vi "UpdateLimsTestStepAutomation.vi"(7 "step_id":u32, 8 "error in (no error)":errorcluster, 9 "instruction_automation":string, 10 "link_automation":string, 11 "ByteGSAPIBase in":refnum<class "ByteGSAPIBase.lvclass">) -> (0 "error out":errorcluster, 2 "Result Step":T1, 3 "ByteGSAPIBase out":refnum<class "ByteGSAPIBase.lvclass">)   [LabVIEW 2019, in "ByteGSWebAPI.lvlib" / "ByteGSAPIBase.lvclass"]
doc: "Update dei dati di automazione"
uses:
  ByteGSAPIBase.lvclass
  TypeDef/UpdateLimsTestStepData.ctl
  ByteGSAPIBase.lvclass/ByteGSAPIBase.ctl
  <vilib>/Bytelabs/ByteREST/ByteRESTClass/ByteRESTBase/RESTBase.lvclass
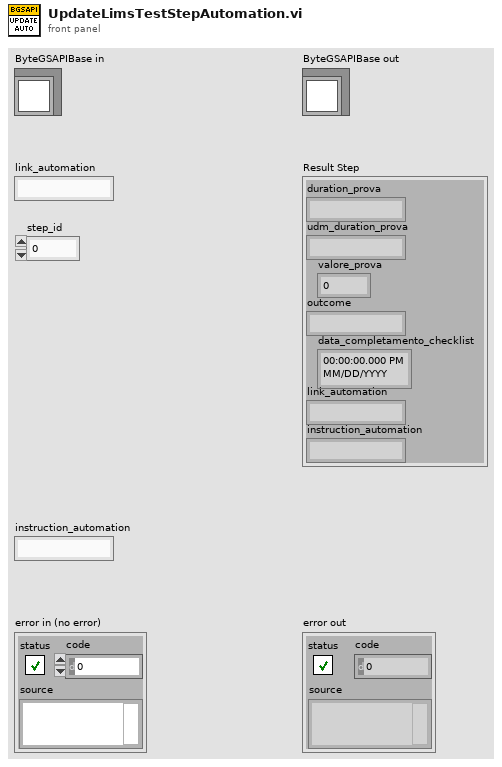
[diagram p1: front panel]
types:
  T1 = typedef "UpdateLimsTestStepData.ctl" = cluster{"duration_prova":string, "udm_duration_prova":string, "valore_prova":dbl, "outcome":string, "data_completamento_checklist":timestamp, "link_automation":string, "instruction_automation":string}
  T2 = cluster{"link_automation":string, "instruction_automation":string, "udm_duration_prova":string, "outcome":string}
  T3 = cluster{"duration_prova":string, "udm_duration_prova":string, "valore_prova":dbl, "outcome":string, "data_completamento_checklist":timestamp, "link_automation":string, "instruction_automation":string}
  T4 = cluster{"duration_prova":string, "udm_duration_prova":string, "data_completamento_checklist":string, "valore_prova":dbl, "outcome":string, "link_automation":string, "instruction_automation":string}
  T5 = typedef "ByteGSWebAPI.lvlib/ByteGSAPIBase.lvclass/Step.ctl" = cluster{"id":i32, "descrizione":string, "prova":string, "assets":T6[], "criterio_accettazione":string, "valore_criterio_accettazione_max":dbl, "valore_criterio_accettazione_min":dbl, "udm_criterio_accettazione":string, "duration_prova":string, "udm_duration_prova":string, "valore_prova":dbl, "outcome":string, "ordine":i32, "user":i32, "link_automation":string, "instruction_automation":string, "data_completamento_checklist":timestamp}
  T6 = typedef "ByteGSWebAPI.lvlib/ByteGSAPIBase.lvclass/Asset.ctl" = cluster{"descrizione":string, "slug":string, "id":i32}
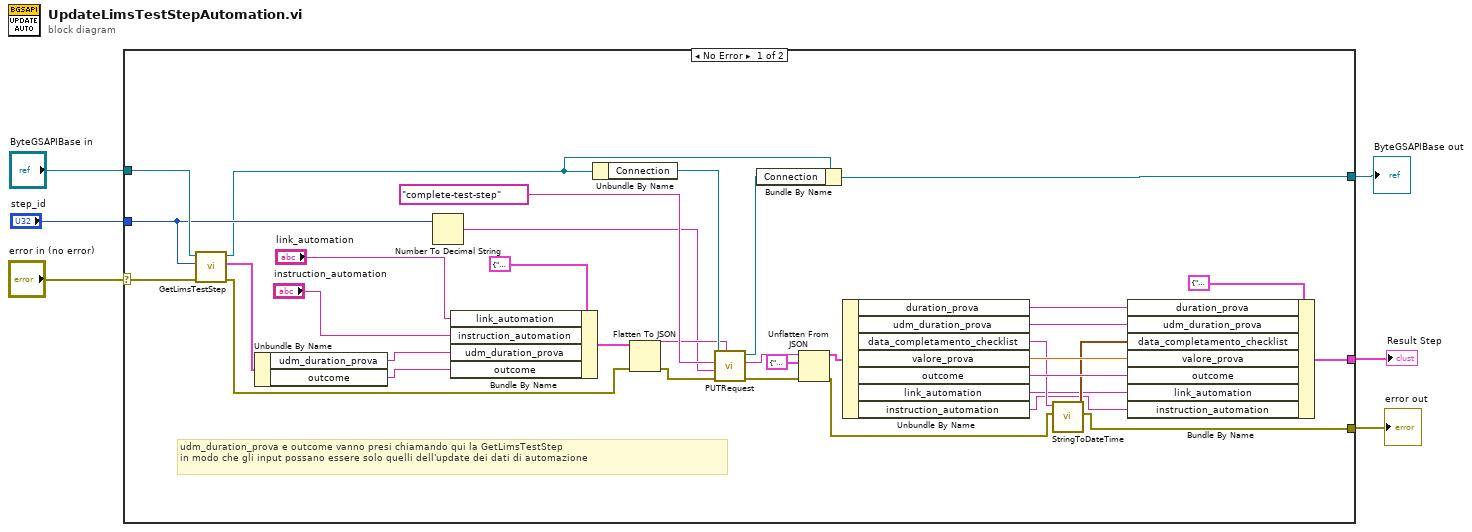
[diagram p0: block diagram]
diagram:
  n1 = case shown="No Error" "error in (no error)" {
    selector: "error in (no error)" -> [w12 w43]
    tunnel: [w24 w43] -> w5
    tunnel: [w40 w42] -> w3
    tunnel: "ByteGSAPIBase in" -> [w14 w42]
    tunnel: [w23 _] -> w2
    tunnel: "step_id" -> [w13 _]
    frame No Error {
      # "udm_duration_prova e outcome vanno presi chiamando qui la GetLimsTestStep\nin modo che gli input possano essere solo quelli dell'update dei dati di automazione"
      n2 = call-dynamic "GetLimsTestStep.vi"("error in (no error)"=w12, "Step-id"=w13, "ByteGSAPIBase in"=w14) -> ("error out"=w11:errorcluster, "StepList"=w9:T5, "ByteGSAPIBase out"=w10:refnum<class "ByteGSAPIBase.lvclass">)  [unwired: 6 in]
      n3 = Unbundle By Name(w9) -> ("udm_duration_prova"=w8:string, "outcome"=w7:string)
      n4 = Number To Decimal String(number=w13) -> (decimal integer string=w17:string)  [unwired: 1 in]
      n5 = Bundle By Name(cluster=T2 {"link_automation"="", "instruction_automation"="", "udm_duration_prova"="", "outcome"=""}, "link_automation"="link_automation", "instruction_automation"="instruction_automation", "udm_duration_prova"=w8, "outcome"=w7) -> (w21:T2)
      n6 = Unbundle By Name(w10) -> ("Connection"=w41:refnum<class "RESTBase.lvclass">)
      n7 = Flatten To JSON(anything=w21, error in (no error)=w11) -> (JSON string=w37:string, 11:w36:errorcluster)  [unwired: 1 in]
      n8 = call-dynamic "PUTRequest.vi"("Body in"=w37, "error in (no error)"=w36, "Parameter"=w17, "Request"="complete-test-step", "ByteRESTBase in"=w41) -> ("error out"=w34:errorcluster, "Body"=w35:string, "ByteRESTBase out"=w39:refnum<class "RESTBase.lvclass">)  [unwired: 3 in, 1 out]
      n9 = Bundle By Name(cluster=w10, "Connection"=w39) -> (w40:refnum<class "ByteGSAPIBase.lvclass">)
      n10 = Unflatten From JSON(JSON string=w35, type and defaults=T4 {"duration_prova"="", "udm_duration_prova"="", "data_completamento_checklist"="", "valore_prova"=0.0, "outcome"="P", "link_automation"="", "instruction_automation"=""}, error in (no error)=w34) -> (value=w32:T4, error out=w20:errorcluster)  [unwired: 4 in]
      n11 = Unbundle By Name(w32) -> ("duration_prova"=w30:string, "udm_duration_prova"=w29:string, "data_completamento_checklist"=w26:string, "valore_prova"=w28:dbl, "outcome"=w27:string, "link_automation"=w19:string, "instruction_automation"=w18:string)
      n12 = call "StringToDateTime.vi"("error in (no error)"=w20, "datetime string"=w26) -> ("error out"=w24:errorcluster, "timestamp"=w25:timestamp)  [unwired: 8 in]
      n13 = Bundle By Name(cluster=T3 {"duration_prova"="", "udm_duration_prova"="", "valore_prova"=0.0, "outcome"="P", "data_completamento_checklist"=timestamp(0 s since 1904-01-01), "link_automation"="", "instruction_automation"=""}, "duration_prova"=w30, "udm_duration_prova"=w29, "data_completamento_checklist"=w25, "valore_prova"=w28, "outcome"=w27, "link_automation"=w19, "instruction_automation"=w18) -> (w23:T3)
    }
    frame Error {
    }
  }
  "error out" <- w5
  "ByteGSAPIBase out" <- w3
  "Result Step" <- w2
